vi "编码规则.vi"(8 "错误输入":errorcluster, 9 "编码正则表达式":string, 11 "功能":enum16{"读取", "写入"}(ring)) -> (0 "错误输出":errorcluster, 2 "正则表达式输出（多行）":string[](array[string]), 3 "正则表达式输出（单行）":string)   [LabVIEW 2020]
uses:
  Global_Variable/Global.vi
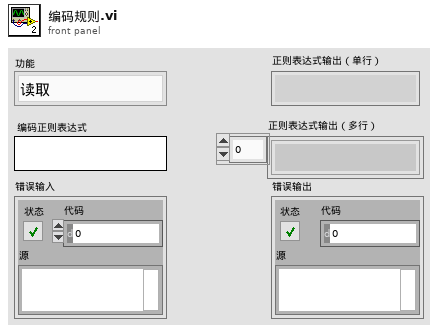
[diagram p1: front panel]
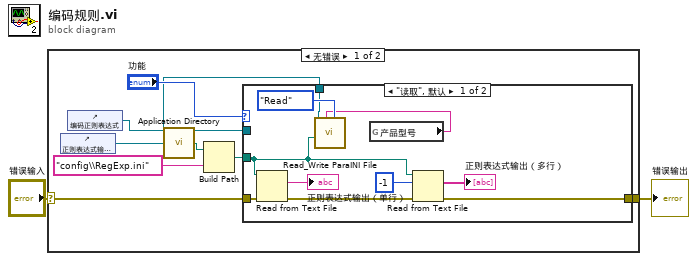
[diagram p0: block diagram]
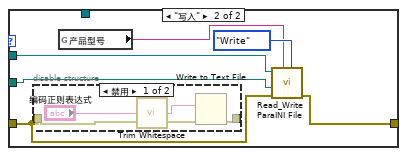
[diagram p2: hidden frame]
diagram:
  n1 = case shown="无错误" "错误输入" {
    selector: "错误输入" -> [w9 w31]
    tunnel: [w8 w31] -> w1
    frame No Error {
      n2 = control-ref of="正则表达式输出（单行）"() -> (w3:refnum<vi>)
      n3 = control-ref of="编码正则表达式"() -> (w4:refnum<vi>)
      n4 = call <vilib>:"Application Directory.vi"() -> ("Application Directory"=w5:path)
      n5 = Build Path(base path=w5, name or relative path="config\\RegExp.ini" ("名称或相对路径")) -> (appended path=w6:path)
      n6 = case shown="\"读取\", 默认" "功能" {
        tunnel: w6 -> [w13 w25]
        tunnel: w9 -> [w19 w23]
        tunnel: [w17 w22] -> w8
        tunnel: w4 -> [_ w24]
        tunnel: w3 -> [w12 _]
        frame "读取", Default {
          n7 = Read from Text File(file (use dialog)=w13, error in=w19) -> (text=→"正则表达式输出（单行）":string, error out=w18:errorcluster)  [unwired: 2 in, 2 out]
          n8 = global read "Global.vi" "产品型号"() -> (w11:string)
          n9 = call "Read_Write ParaINI File.vi"("Mode"=enum16{"Read", "Write"}."Read", "Section"=w11, "Filepath"=w13, "Ctl Refnum"=w12) -> ()  [unwired: 7 in, 1 out]
          n10 = Read from Text File ("读取文本文件")(file (use dialog)=w13, count=-1 ("计数"), error in=w18) -> (text=→"正则表达式输出（多行）":string[], error out=w17:errorcluster)  [unwired: 1 in, 2 out]
        }
        frame "写入" {
          n11 = disable-structure shown="禁用" {
            disable-tunnel: w23 -> [w29 _]
            disable-tunnel: [w28 _] -> _
            frame Disabled {
              n12 = call <vilib>:"Trim Whitespace.vi"("string"="编码正则表达式") -> ("trimmed string"=w30:string)  [unwired: 1 in]
              n13 = Write to Text File(text=w30, error in=w29) -> (error out=w28:errorcluster)  [unwired: 2 in, 2 out]
            }
            frame Enabled {
            }
          }
          n14 = global read "Global.vi" "产品型号"() -> (w21:string)
          n15 = call "Read_Write ParaINI File.vi"("Mode"=enum16{"Read", "Write"}."Write", "Section"=w21, "error in"=w23, "Filepath"=w25, "Ctl Refnum"=w24) -> ("error out"=w22:errorcluster)  [unwired: 6 in]
        }
      }
    }
    frame Error {
    }
  }
  "错误输出" <- w1
